vi "数据记录按钮.vi"() -> ()   [LabVIEW 2014]
panel:
  in  "清空记录":bool
  out "状态":string
  out "记录":string
  out "数值":i32
  in  "退出":bool
  in  "记录":bool
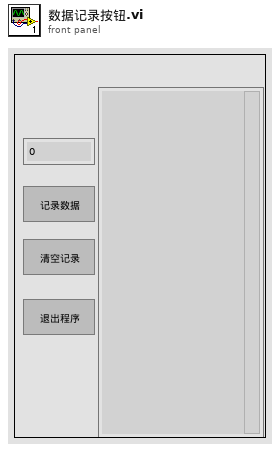
[diagram p1: front panel]
types:
  T1 = enum16{"open", "replace", "create", "open or create", "replace or create", "replace or create with confirmation"}
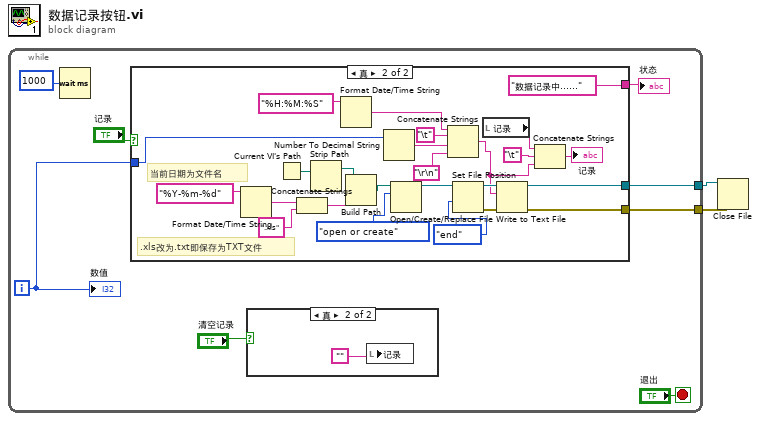
[diagram p0: block diagram]
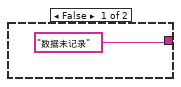
[diagram p3: hidden frame]
diagram:
  n1 = while {
    tunnel: [w5] -> w2
    tunnel: [w6] -> w1
    i -> [w7]
    stop <- "退出" stop-if-true
    n2 = Wait (ms)(milliseconds to wait=u32 1000 ("等待时间（毫秒）")) -> ()  [unwired: 1 out]
    n3 = case shown="真" "记录" {
      tunnel: w7 -> [_ w37]
      tunnel: [_ w18] -> w5
      tunnel: [_ w36] -> w6
      tunnel: ["数据未记录" "数据记录中……"] -> w4
      frame False {
      }
      frame True {
        # ".xls改为.txt即保存为TXT文件"
        # "当前日期为文件名"
        n4 = Format Date/Time String(time format string (%c)="%Y-%m-%d" ("时间格式字符串(%c)")) -> (date/time string=w27:string)  [unwired: 2 in]
        n5 = Current VI's Path() -> (path=w25:path)
        n6 = Concatenate Strings(w27, ".xls" ("名称或相对路径")) -> (w30:string)
        n7 = Strip Path(path=w25) -> (stripped path=w26:path)  [unwired: 1 out]
        n8 = Format Date/Time String(time format string (%c)="%H:%M:%S" ("时间格式字符串(%c)")) -> (date/time string=w14:string)  [unwired: 2 in]
        n9 = Build Path(base path=w26, name or relative path=w30) -> (appended path=w32:path)
        n10 = Number To Decimal String(number=w37) -> (decimal integer string=w35:string)  [unwired: 1 in]
        n11 = Open/Create/Replace File(file path (use dialog)=w32, operation (0:open)=T1."open or create" ("操作(0:open)")) -> (refnum out=w29:refnum<file>)  [unwired: 4 in, 2 out]
        n12 = Concatenate Strings(w14, "\t", w35, "\r\n") -> (w19:string)
        n13 = Set File Position(refnum=w29, from (0:start)=enum16{"start", "end", "current"}."end" ("自（0:起始）")) -> (refnum out=w24:refnum<file>, error out=w23:errorcluster)  [unwired: 2 in]
        n14 = local read "记录"() -> (w21:string)
        n15 = Write to Text File(file (use dialog)=w24, text=w19, error in=w23) -> (refnum out=w18:refnum<file>, error out=w36:errorcluster)  [unwired: 1 in, 1 out]
        n16 = Concatenate Strings(w21, "\t", w19) -> (→"记录":string)
      }
    }
    "状态" <- w4
    n17 = case shown="真" "清空记录" {
      frame False {
      }
      frame True {
        n18 = local write "记录"("") -> ()
      }
    }
    "数值" <- w7
  }
  n19 = Close File(refnum=w2, error in=w1) -> ()  [unwired: 2 out]
